vi "Read Error.vi"(8 "error in (no error)":errorcluster, 11 "AcknowledgeMsg in":refnum<class "CS++AcknowledgeMsg.lvclass">) -> (0 "error out":errorcluster, 2 "Error":errorcluster, 3 "AcknowledgeMsg out":refnum<class "CS++AcknowledgeMsg.lvclass">)   [LabVIEW 2015, in "CS++AcknowledgeMsg.lvlib" / "CS++AcknowledgeMsg.lvclass"]
uses:
  CS++AcknowledgeMsg.lvclass
  CS++AcknowledgeMsg.lvclass/CS++AcknowledgeMsg.ctl
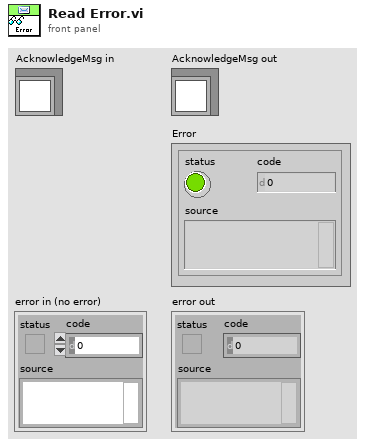
[diagram p1: front panel]
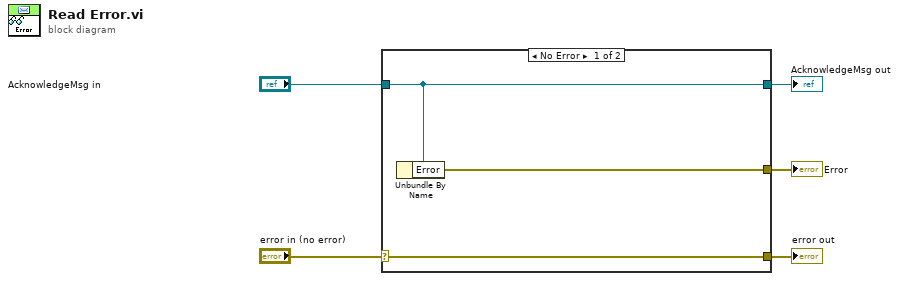
[diagram p0: block diagram]
diagram:
  n1 = case shown="No Error" "error in (no error)" {
    selector: "error in (no error)" -> [w8 w9]
    tunnel: [w8 w9] -> w4
    tunnel: [w7 w10] -> w2
    tunnel: "AcknowledgeMsg in" -> [w7 w10]
    tunnel: [w6 _] -> w1
    frame No Error {
      n2 = Unbundle By Name(w7) -> ("Error"=w6:errorcluster)
    }
    frame Error {
    }
  }
  "error out" <- w4
  "AcknowledgeMsg out" <- w2
  "Error" <- w1
